vi "P4CMD_Sup SCC Convert EOL to LF.vi"(2 "input string":string) -> (0 "output string":string)   [LabVIEW 2020, in "NI_SCC_P4CMD.lvlib"]
uses:
  <vilib>/SourceControl/Providers/P4CMD/NI_SCC_P4CMD.lvlib
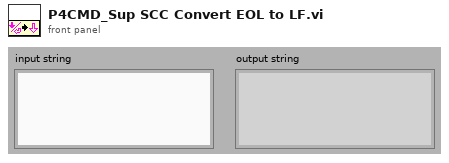
[diagram p1: front panel]
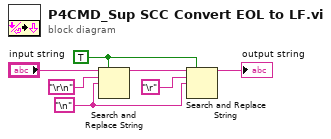
[diagram p0: block diagram]
diagram:
  w3 = "\n" ("Line Feed Constant")
  w4 = TRUE ("replace all? (F)")
  n1 = Search and Replace String(replace all?=w4, input string="input string", search string="\r\n" ("End of Line Constant"), replace string=w3) -> (result string=w6:string)  [unwired: 4 in, 3 out]
  n2 = Search and Replace String(replace all?=w4, input string=w6, search string="\r" ("Carriage Return Constant"), replace string=w3) -> (result string=→"output string":string)  [unwired: 4 in, 3 out]
